vi "FPGA_Main.vi"() -> ()   [LabVIEW 2017]
uses:
  <vilib>/Platform/TimedLoop/XDataNode/timing_clust.ctl
  <vilib>/Platform/TimedLoop/XDataNode/nitl_modes.ctl
  <vilib>/Platform/TimedLoop/XDataNode/wakeup.ctl
  <vilib>/rvi/Analysis/measure/FFT/simModelSupport/niFPGA FFT Sim Properties.ctl
  <vilib>/rvi/Analysis/measure/FFT/simModelSupport/niFPGA FFT Sim Types.ctl
  <vilib>/rvi/Analysis/measure/FFT/simModelSupport/niFpgaFFTSimArithmeticProperties.ctl
  <vilib>/rvi/Analysis/measure/FFT/simModelSupport/niFpgaFFTSimDfxp.ctl
  <vilib>/fxp/LVFixedPointQuantizationPolicyTypeDef.ctl
  <vilib>/rvi/FXPMathLib/FxpRectToPolar/subVIs/nifxpmath_RectToPolar_SimConfig.ctl
  <vilib>/rvi/FXPMathLib/FxpDiv/subVIs/nifxpmath_Div_SimConfig.ctl
  <vilib>/rvi/Emulation/niFpgaSctlEmulationGetInTimedLoop.vi
  <vilib>/rvi/Emulation/niFpgaProcessEmulError.vi
  <vilib>/rvi/Emulation/niFpgaEmulationReportErrorSimple.vi
  <vilib>/rvi/Emulation/niFpgaGetClockAttributes.vi
  <vilib>/rvi/Emulation/niFpgaCriticalErrorInLSC.vi
  <vilib>/rvi/Emulation/niFpgaEmulationIsFPGAContextNoSignature.vi
  <vilib>/rvi/errors/niFpgaSetErrorForExecOnDevCompSimple.vi
  <vilib>/rvi/eio/common/nirviEmuReportErrorAndStop.vi
  <vilib>/rvi/DataTransferAndStorage/Container/Common/niFpgaContainerGetUniqueNameForEmu.vi
  <vilib>/rvi/FIFO/Fifo_Resource/nirvififoEmulationSetSize.vi
  <vilib>/rvi/FIFO/Fifo_Resource/nirviFifoEmulationQueueMgr.vi
  <instcachedir>/0/nirviFifoEmulationQueueMgr_E5CAEC123FF24DC58D834DCA3CDAA9B5.lvgen/nirviFifoEmulationQueueMgr_E5CAEC123FF24DC58D834DCA3CDAA9B5_004.vi
  <vilib>/rvi/FIFO/Fifo_Resource/nirvififoEmulationDetermineInputValidOut.vi
  <vilib>/rvi/FIFO/Fifo_Resource/nirvififoEmulationCreateLock.vi
  <vilib>/rvi/FIFO/Fifo_Resource/nirvififoEmulationObtainLock.vi
  <vilib>/rvi/FIFO/Fifo_Resource/nirvififoEmulationReleaseLock.vi
  <vilib>/rvi/occurrence/nirviWaitOnOccurrenceBase.vi
  <vilib>/rvi/errors/nirviReportUnexpectedCaseInternalError.vi
  <vilib>/rvi/errors/nirviReportUnexpectedCaseInternalError (U32).vi
  <vilib>/rvi/eio/common/nirviEmuTemplateMethod_errors.vi
  <instcachedir>/0/nirviFifoEmulationQueueMgr_E5CAEC123FF24DC58D834DCA3CDAA9B5.lvgen/nirviFifoEmulationQueueMgr_E5CAEC123FF24DC58D834DCA3CDAA9B5_005.vi
  <vilib>/Utility/error.llb/Clear Errors.vi
  <vilib>/rvi/Analysis/common/codeGenErrors/XNode/niFpgaXNodeCodeGenErrorHandle.vi
  <vilib>/rvi/interface/RandomDataEmulation/niFpgaRandomDataHandleErrors.vi
  <vilib>/rvi/Memory/Memory_Emulation/niFpgaMemoryEmulationCacheClearOnFirstRun.vi
  <vilib>/rvi/Memory/Memory_Emulation/nirvimemoryEmulationManagerCache_MakeExclusive.vi
  <vilib>/rvi/Memory/Memory_Emulation/niFpgaMemoryEmulationValidateCache.vi
  <vilib>/rvi/Memory/Memory_Emulation/nirvimemoryEmulationManagerCache_InsertValue.vi
  <vilib>/rvi/Memory/Memory_Emulation/nirvimemoryEmulationManagerCache_ReleaseExclusive.vi
  <vilib>/rvi/Memory/Memory_Emulation/nirvimemoryEmulationManagerCache_GetValue.vi
  <vilib>/rvi/Memory/Memory_Emulation/nirvimemoryEmulationManagerCache_SetValue.vi
  <vilib>/rvi/DataTransferAndStorage/Container/Common/niFpgaContainerExecOnDevCompGetState.vi
  <vilib>/rvi/Analysis/measure/FFT/simModelSupport/niFpgaFFTSimModelCore.vi
  <vilib>/rvi/FXPMathLib/FxpRectToPolar/simVIs/DllFxpRectToPolarTemp_sub.vi
  <vilib>/rvi/FXPMathLib/FxpDiv/simVIs/DllFxpDivTemp_sub.vi
  <vilib>/Platform/TimedLoop/XDataNode/XDataNode.xnode
  <vilib>/rvi/DataTransferAndStorage/Container/XNode/niFpgaContainer.xnode
  <vilib>/rvi/FIFO/Fifo_Resource/nirvififoEmulationWrite.vi
  <vilib>/eio/EIONode/EIONode.xnode
  <vilib>/rvi/FIFO/Fifo_Resource/nirvififoEmulationRead.vi
  <vilib>/rvi/Analysis/measure/LMRsmpl/XNode/niFPGA Rational Resampler.xnode
  <vilib>/rvi/interface/RandomDataEmulation/nirviRandomDataFpgaReadWriteTemplate.vi
  <vilib>/rvi/DataTransferAndStorage/Register/Emulation/niFpgaRegisterEmulation.vi
  <vilib>/rvi/FIFO/Fifo_Resource/niFpgaFifoEmulationRefIn.vi
  <vilib>/rvi/Analysis/measure/window/XNode/niFPGA Scaled Window.xnode
  <vilib>/rvi/FXPMathLib/basic elements/FxpDiscreteDelay/XNode/nifxpmath_DiscreteDelay.xnode
  <vilib>/rvi/FXPMathLib/FxpMul/XNode/nifxpmath_Multiplier.xnode
  <vilib>/rvi/Analysis/measure/FFT/XNode/niFpgaFFT.xnode
  <vilib>/rvi/FXPMathLib/FxpRectToPolar/XNode/nifxpmath_RectToPolar.xnode
  <vilib>/rvi/FXPMathLib/FxpDiv/XNode/nifxpmath_Div.xnode
  <vilib>/Platform/TimedLoop/XDataNode/XDNodeRunTimeDep.lvlib
  <vilib>/rvi/FXPMathLib/sim/FxpSim.dll
panel:
  in  "DC":fxp<+/-,12,9>=127.5
  in  "Windows in Average":u32=2
  out "ButtonPressed?":bool
  in  "LED States":u8=3
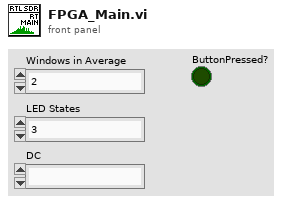
[diagram p1: front panel]
types:
  T1 = typedef "XDNodeRunTimeDep.lvlib/timing_clust.ctl" = cluster{"Expected End [f-1]":u64, "Actual End [f-1]":u64, "Finished Late? [f-1]":bool, "Expected End [i-1]":u64, "Actual End [i-1]":u64, "Finished Late? [i-1]":bool, "Expected Start [i]":u64, "Actual Start [i]":u64, "Expected Start [f]":u64, "Actual Start [f]":u64, "Source Name":string, "Structure Name":string, "Period":i64, "Deadline":i64, "Offset":i64, "Start":i64, "Priority":i32, "Timeout":i32, "Mode":T2, "Wakeup Reason":T3, "Error":errorcluster, "Source Type":string, "Secondary Source Type":string, "Global End Time":u64, "Global Start Time":u64, "Frame Duration":u64, "Iteration Duration":u64, "Assigned CPU":i32, "I/O Scan Engine Mode":u32}
  T2 = typedef "XDNodeRunTimeDep.lvlib/nitl_modes.ctl" = enum32{"No Change", "Process missed periods, maintain original phase", "Discard missed periods, maintain original phase", "Process missed periods, ignore original phase", "Discard missed periods, ignore original phase"}
  T3 = typedef "XDNodeRunTimeDep.lvlib/wakeup.ctl" = enum32{"Normal", "Aborted", "Asynchronous wakeup", "Timing source error", "Timed loop error", "Timeout"}
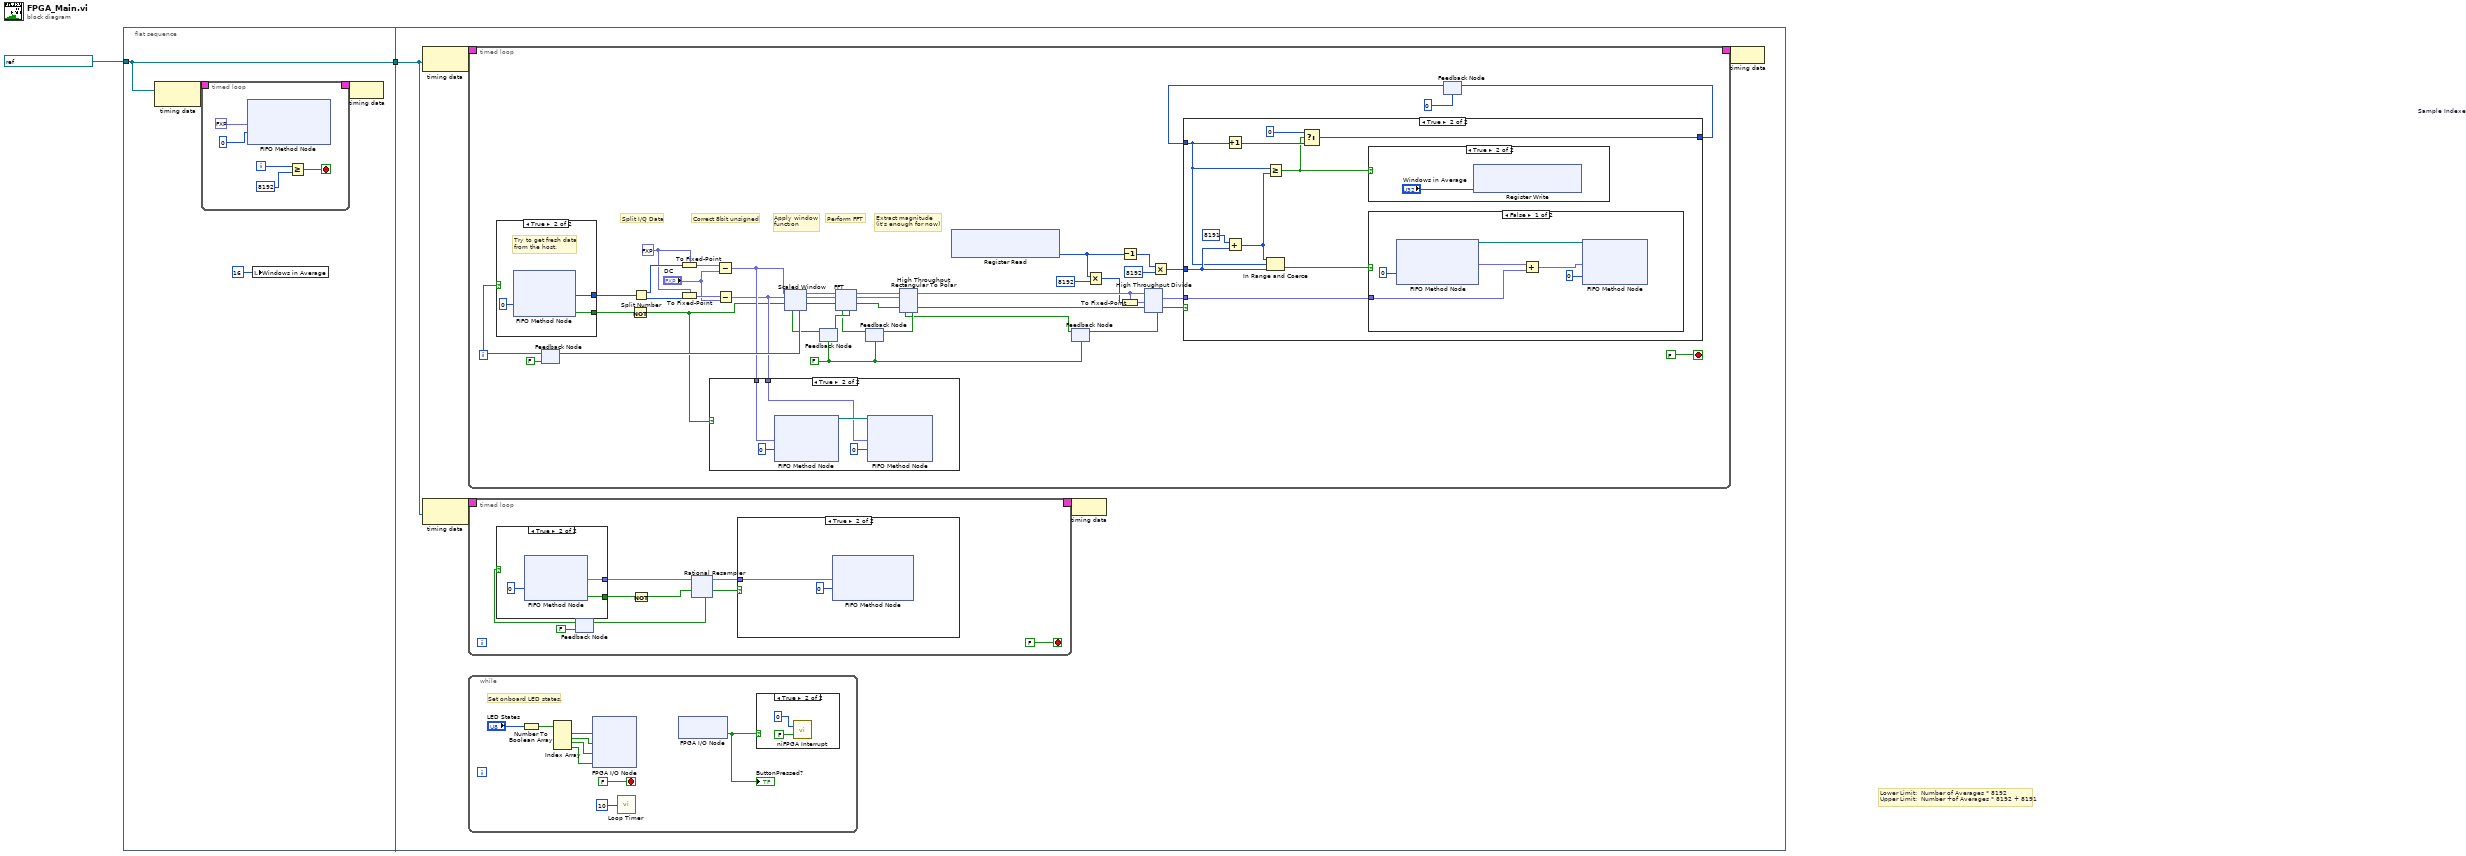
[diagram p0: block diagram]
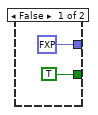
[diagram p2: hidden frame]
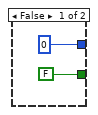
[diagram p5: hidden frame]
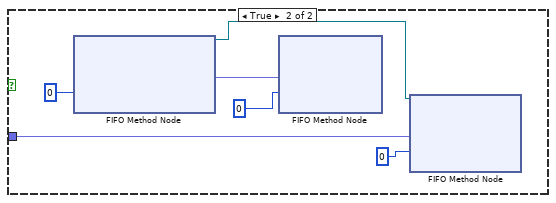
[diagram p8: hidden frame]
diagram:
  # "Lower Limit:  Number of Averages * 8192\nUpper Limit:  Number +of Averages * 8192 + 8191"
  n1 = flat-sequence {
    tunnel: refnum<k21> "40 MHz Onboard Clock" ("Source Name") -> [w4]
    tunnel: [w4] -> w1
    tunnel: w1 -> [w18]
    frame #0 {
      n2 = node-c288(w4) -> (w6:T1)
      n3 = timed-loop {
        timing: w6 -> [_]
        timing-out: [_] -> w5
        i -> [w8]
        stop <- w9 stop-if-true
        n4 = xnode ("FIFO Method Node")("Element"=fxp<+,32,8> 0.0, "Timeout"=0) -> ()  [unwired: 1 in, 2 out]
        n5 = Greater Or Equal?(x=w8, y=8192) -> (x >= y?=w9:bool)
      }
      n6 = local write "Windows in Average"(u32 16 ("Windows in Average")) -> ()
      n7 = node-c288(w5) -> ()
    }
    frame #1 {
      n8 = node-c288(w18) -> (w22:T1)
      n9 = node-c288(w18) -> (w20:T1)
      n10 = timed-loop {
        timing: w22 -> [_]
        timing-out: [_] -> w21
        stop <- FALSE stop-if-true
        w131 = fxp<+/-,12,9> 0.0 ("fixed-point type")
        w143 = FALSE ("ready for input")
        # "Correct 8bit unsigned"
        # "Extract magnitude\n(it's enough for now)"
        # "Perform FFT"
        # "Apply window\nfunction"
        # "Split I/Q Data"
        n11 = feedback #1(FALSE ("ready for input")) -> (w138:bool)
        n12 = case shown="True" w138 {
          tunnel: [u16 0 ("Element") w168] -> w142
          tunnel: [FALSE ("Timed Out?") w167] -> w155
          frame False {
          }
          frame True {
            # "Try to get fresh data\nfrom the host."
            n13 = xnode ("FIFO Method Node")("Timeout"=0) -> ("Element"=w168:u16, "Timed Out?"=w167:bool)  [unwired: 1 in, 1 out]
          }
        }
        n14 = Not(x=w155) -> (.not. x?=w119:bool)
        n15 = Split Number(x=w142) -> (hi(x)=w141:u8, lo(x)=w135:u8)
        n16 = To Fixed-Point(fixed-point type=w131, number=w141) -> (fixed-point=w140:fxp<+/-,12,9>)
        n17 = To Fixed-Point(fixed-point type=w131, number=w135) -> (fixed-point=w136:fxp<+/-,12,9>)
        n18 = Subtract(x=w140, y="DC") -> (x-y=w121:fxp<+/-,13,10>)
        n19 = Subtract(x=w136, y="DC") -> (x-y=w120:fxp<+/-,13,10>)
        n20 = case shown="True" w119 {
          tunnel: w121 -> [_ w164]
          tunnel: w120 -> [_ w160]
          frame False {
          }
          frame True {
            n21 = xnode ("FIFO Method Node")("Element"=w164, "Timeout"=0) -> ("FIFO Out"=w163:refnum<k21>)  [unwired: 1 in, 1 out]
            n22 = xnode ("FIFO Method Node")("Element"=w160, "Timeout"=0, "FIFO In"=w163) -> ()  [unwired: 2 out]
          }
        }
        n23 = feedback #2(w143) -> (w151:bool)
        n24 = xnode "Scaled Window"("real data in"=w121, "imaginary data in"=w120, "input valid"=w119, "ready for output"=w151) -> ("real data out"=w139:fxp<+/-,15,12>, "imaginary data out"=w158:fxp<+/-,15,12>, "output valid"=w154:bool, "ready for input"=w153:bool)  [unwired: 1 out]
        n25 = feedback-in #1(w153) -> ()
        n26 = feedback #3(w143) -> (w149:bool)
        n27 = xnode "FFT"("real data in"=w139, "imaginary data in"=w158, "input valid"=w154, "ready for output"=w149) -> ("ready for input"=w152:bool, "real data out"=w157:fxp<+/-,29,26>, "imaginary data out"=w156:fxp<+/-,29,26>, "output valid"=w132:bool)  [unwired: 1 in, 1 out]
        n28 = feedback-in #2(w152) -> ()
        n29 = xnode ("Register Read")() -> ("Data"=w122:u32)  [unwired: 1 in, 1 out]
        n30 = feedback #4(w143) -> (w144:bool)
        n31 = xnode "High Throughput Rectangular To Polar"("x"=w157, "y"=w156, "input valid"=w132, "ready for output (T)"=w144) -> ("magnitude"=w148:fxp<+,29,26>, "output valid"=w146:bool, "ready for input"=w150:bool)  [unwired: 1 out]
        n32 = feedback-in #3(w150) -> ()
        n33 = Multiply(x=w122, y=u32 8192) -> (x*y=w126:u32)
        n34 = Decrement(x=w122) -> (x-1=w123:u32)
        n35 = To Fixed-Point(fixed-point type=w148, number=w126) -> (fixed-point=w147:fxp<+,29,26>)
        n36 = xnode "High Throughput Divide"("x"=w148, "y"=w147, "input valid"=w146) -> ("x/y"=w134:fxp<+,32,5>, "output valid"=w133:bool, "ready for input"=w145:bool)  [unwired: 1 in]
        n37 = feedback-in #4(w145) -> ()
        n38 = Multiply(x=w123, y=u32 8192) -> (x*y=w124:u32)
        n39 = feedback #5 "Sample Indexer"(u32 0) -> (w128:u32)
        n40 = case shown="True" w133 {
          tunnel: w134 -> [_ w320]
          tunnel: w128 -> [w310 w312]
          tunnel: [w310 w316] -> w129
          tunnel: w124 -> [_ w318]
          frame False {
          }
          frame True {
            n41 = Increment(x=w312) -> (x+1=w314:u32)
            n42 = Add(x=u32 8191, y=w318) -> (x+y=w313:u32)
            n43 = Greater Or Equal?(x=w312, y=w313) -> (x >= y?=w311:bool)
            n44 = In Range and Coerce(upper limit=w313, x=w312, lower limit=w318) -> (In Range?=w319:bool)  [unwired: 1 out]
            n45 = Select(t=u32 0, s=w311, f=w314) -> (s? t:f=w316:u32)
            n46 = case shown="True" w311 {
              frame False {
              }
              frame True {
                n47 = xnode ("Register Write")("Data"="Windows in Average") -> ()  [unwired: 1 in, 1 out]
              }
            }
            n48 = case shown="False" w319 {
              tunnel: w320 -> [w327 w330]
              frame False {
                n49 = xnode ("FIFO Method Node")("Timeout"=0) -> ("Element"=w326:fxp<+,32,5>, "FIFO Out"=w322:refnum<k21>)  [unwired: 1 in, 1 out]
                n50 = Add(x=w326, y=w327) -> (x+y=w324:fxp<+,32,5>)
                n51 = xnode ("FIFO Method Node")("Element"=w324, "Timeout"=0, "FIFO In"=w322) -> ()  [unwired: 2 out]
              }
              frame True {
                n52 = xnode ("FIFO Method Node")("Timeout"=0) -> ("Element"=w332:fxp<+,32,5>, "FIFO Out"=w328:refnum<k21>)  [unwired: 1 in, 1 out]
                n53 = xnode ("FIFO Method Node")("Element"=w332, "Timeout"=0) -> ()  [unwired: 1 in, 2 out]
                n54 = xnode ("FIFO Method Node")("Element"=w330, "Timeout"=0, "FIFO In"=w328) -> ()  [unwired: 2 out]
              }
            }
          }
        }
        n55 = feedback-in #5(w129) -> ()
      }
      n56 = timed-loop {
        timing: w20 -> [_]
        timing-out: [_] -> w19
        stop <- FALSE stop-if-true
        n57 = feedback #6(FALSE ("ready for input")) -> (w24:bool)
        n58 = case shown="True" w24 {
          tunnel: [fxp<+/-,11,10> 0.0 ("Element") w36] -> w30
          tunnel: [TRUE ("Timed Out?") w34] -> w29
          frame False {
          }
          frame True {
            n59 = xnode ("FIFO Method Node")("Timeout"=0) -> ("Element"=w36:fxp<+/-,13,10>, "Timed Out?"=w34:bool)  [unwired: 1 in, 1 out]
          }
        }
        n60 = Not(x=w29) -> (.not. x?=w28:bool)
        n61 = xnode "Rational Resampler"("input data"=w30, "input valid"=w28) -> ("output data"=w26:fxp<+/-,15,10>, "output valid"=w27:bool, "ready for input"=w25:bool)  [unwired: 1 in, 1 out]
        n62 = feedback-in #6(w25) -> ()
        n63 = case shown="True" w27 {
          tunnel: w26 -> [_ w38]
          frame False {
          }
          frame True {
            n64 = xnode ("FIFO Method Node")("Element"=w38, "Timeout"=0) -> ()  [unwired: 1 in, 2 out]
          }
        }
      }
      n65 = while {
        stop <- FALSE stop-if-true
        # "Set onboard LED states."
        n66 = Number To Boolean Array(number="LED States") -> (Boolean array=w377:bool[])
        n67 = Index Array(array=w377) -> (element #1=w376:bool, element #2=w375:bool, element #3=w374:bool, element #4=w373:bool)  [unwired: 4 in]
        n68 = xnode "FPGA I/O Node"("LED0"=w376, "LED1"=w375, "LED2"=w374, "LED3"=w373) -> ()  [unwired: 4 in, 4 out]
        n69 = call "Loop Timer"("Count(mSec)"=u8 10) -> ()  [unwired: 1 out]
        n70 = xnode "FPGA I/O Node"() -> ("Button0"=w370:bool)  [unwired: 1 in, 1 out]
        "ButtonPressed?" <- w370
        n71 = case shown="True" w370 {
          frame False {
          }
          frame True {
            n72 = call <vilib>:"niFPGA Interrupt.vi"("Wait Until Cleared (F)"=FALSE, "IRQ Number (0)"=u8 0) -> ()  [unwired: 1 in]
          }
        }
      }
      n73 = node-c288(w19) -> ()
      n74 = node-c288(w21) -> ()
    }
  }
